vi "LabVIEW_GUI.vi"() -> ()   [LabVIEW 2025]
uses:
  subs/PIV_params.ctl
  subs/PIV_postParameters.ctl
panel:
  in  "xy scale":dbl=70.0 format="%#_13g"
  in  "Offset":cluster{i32, i32}={10, 500}
  in  "Scaling":cluster{"dt (sec)":dbl, "pixels/mm":dbl}={"dt (sec)"=0.02, "pixels/mm"=96.52}
  in  "post-processing":T1={"mask threshold"=1.02, "method"="localmean", "max iteration"=3, "kernal size"=3}
  in  "PIV params":T2={"t"=path "/Users/crogers/GitHub/ME51-25/PIV/odd_flow/frame_0_delay-0.14s.png", "t + dt"=path "/Users/crogers/GitHub/ME51-25/PIV/odd_flow/frame_1_delay-0.14s.png", "PIV params"={"window size"=32, "search size"=38, "overlap"=17}}
  in  "scale":dbl=5.0 format="%#_13g"
  out "picture":picture
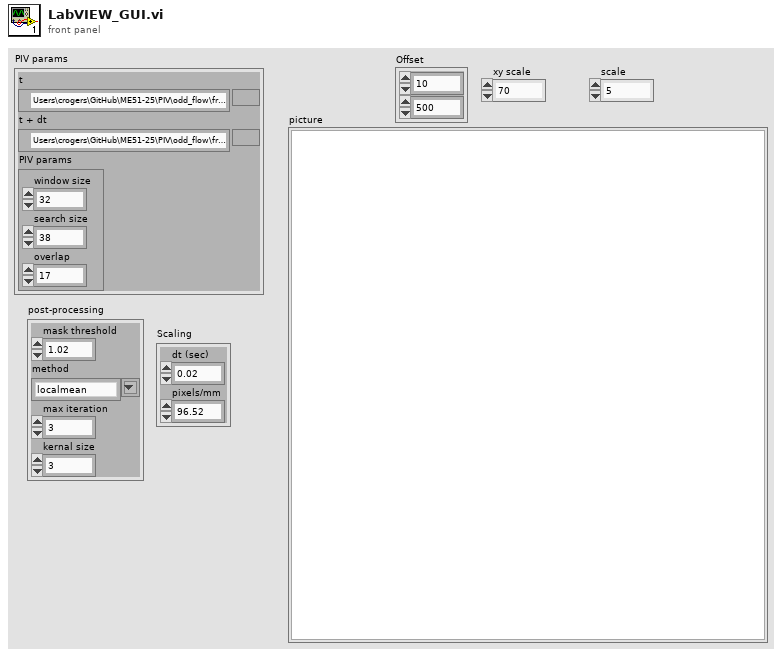
[diagram p1: front panel]
types:
  T1 = typedef "PIV_postParameters.ctl" = cluster{"mask threshold":dbl, "method":string, "max iteration":u8, "kernal size":u8}
  T2 = typedef "PIV_params.ctl" = cluster{"t":path, "t + dt":path, "PIV params":cluster{"window size":i16, "search size":i16, "overlap":i16}}
  T3 = typedef "PIV_velocities.ctl" = cluster{"x":dbl[][], "y":dbl[][], "u":dbl[][], "v":dbl[][], "Sig2noise":dbl[][]}
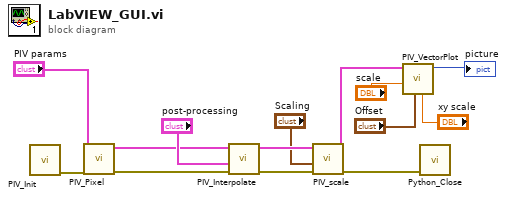
[diagram p0: block diagram]
diagram:
  n1 = call "PIV_Init.vi"() -> ("error out"=w14:errorcluster)  [unwired: 11 in]
  n2 = call "PIV_Pixel.vi"("error in (no error)"=w14, "PIV params"="PIV params") -> ("error out"=w11:errorcluster, "pixels"=w8:T3)  [unwired: 8 in]
  n3 = call "PIV_Interpolate.vi"("error in (no error)"=w11, "post-processing"="post-processing", "raw"=w8) -> ("error out"=w7:errorcluster, "interpolated"=w5:T3)  [unwired: 7 in]
  n4 = call "PIV_scale.vi"("error in (no error)"=w7, "Scaling"="Scaling", "interpolated"=w5) -> ("error out"=w6:errorcluster, "velocities"=w4:T3)  [unwired: 7 in]
  n5 = call "PIV_VectorPlot.vi"("xy scale"="xy scale", "Offset"="Offset", "vector scale"="scale", "velocities"=w4) -> ("vectors"=→"picture":picture)  [unwired: 7 in]
  n6 = call "Python_Close.vi"("error in (no error)"=w6) -> ()  [unwired: 2 in, 1 out]
